vi "LWXPS_PositionerCorrectorSR1AccelerationSet.vi"(0 "Closed loop status":bool, 1 "Proportional gain":dbl, 2 "Integral gain":dbl, 3 "Velocity gain":dbl, 4 "Observer frequency":dbl, 5 "Velocity compensation gain":dbl, 6 "Positioner Name":string, 7 "Acceleration compensation gain":dbl, 8 "XPS Reference IN":refnum<k24>, 9 "Jerk compensation gain":dbl, 11 "LabVIEW error IN":errorcluster) -> (14 "XPS Reference OUT":refnum<k24>, 15 "Returned error code":i32, 16 "XPS Error String":string, 19 "LabVIEW error OUT":errorcluster)   [LabVIEW 2014]
uses:
  D:/XPSQ8_LabView_Library/Development/Source/Dll/Newport.XPS.CommandInterface.dll
  Dll/Newport.XPS.CommandInterface.dll
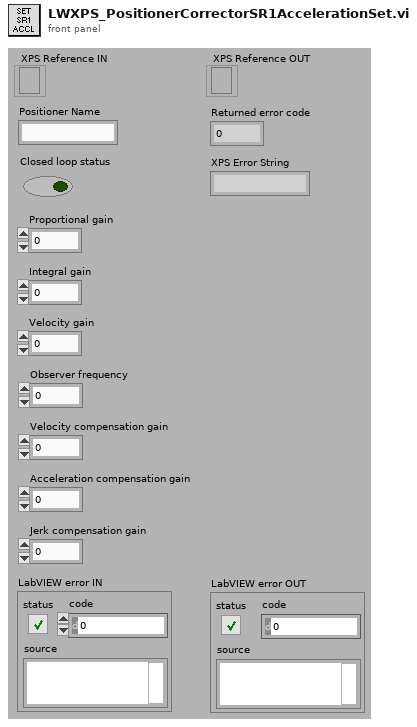
[diagram p1: front panel]
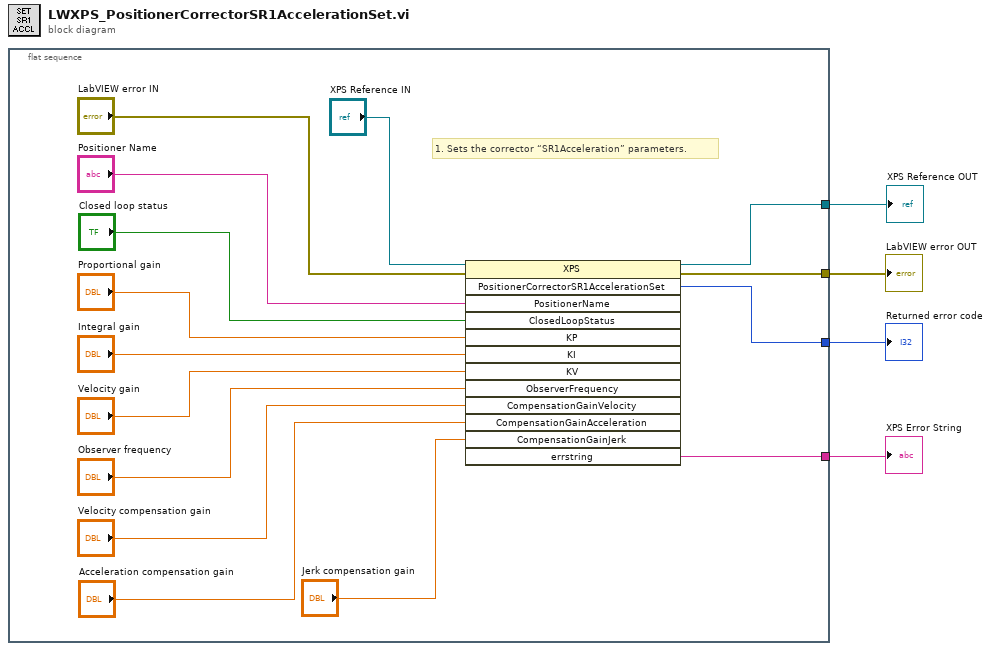
[diagram p0: block diagram]
diagram:
  n1 = flat-sequence {
    tunnel: [w15] -> w4
    tunnel: [w18] -> w3
    tunnel: [w17] -> w2
    tunnel: [w7] -> w1
    frame #0 {
      # "1. Sets the corrector “SR1Acceleration” parameters."
      n2 = invoke class="XPS" method="PositionerCorrectorSR1AccelerationSet"(reference="XPS Reference IN", error in="LabVIEW error IN", "PositionerName"="Positioner Name", "ClosedLoopStatus"="Closed loop status", "KP"="Proportional gain", "KI"="Integral gain", "KV"="Velocity gain", "ObserverFrequency"="Observer frequency", "CompensationGainVelocity"="Velocity compensation gain", "CompensationGainAcceleration"="Acceleration compensation gain", "CompensationGainJerk"="Jerk compensation gain") -> (reference out=w15:refnum<k24>, error out=w18:errorcluster, "PositionerCorrectorSR1AccelerationSet"=w17:i32, "errstring"=w7:string)  [unwired: 2 in, 9 out]
    }
  }
  "XPS Error String" <- w1
  "XPS Reference OUT" <- w4
  "LabVIEW error OUT" <- w3
  "Returned error code" <- w2
